vi "TIFF Read RGBA Image Oriented.vi"(0 "para0":cluster{}, 1 "para4":cluster{}, 5 "para1":cluster{}, 7 "para2":cluster{}, 9 "para3":cluster{}, 11 "error in (no error)":errorcluster, 12 "para5":cluster{}) -> (4 "para0 out":cluster{}, 6 "function return":i32, 10 "para3 out":cluster{}, 15 "error out":errorcluster)   [LabVIEW 2018]
doc: "LIBTIFF_DLL_IMPEXP int TIFFReadRGBAImageOriented(TIFF*, uint32, uint32, uint32*,\n int = ORIENTATION_BOTLEFT, int = 0);"
uses:
  libtiff3.dll
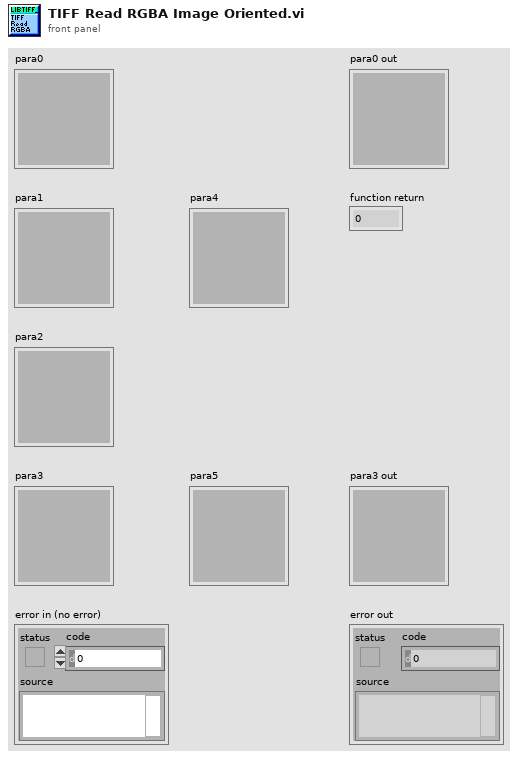
[diagram p1: front panel]
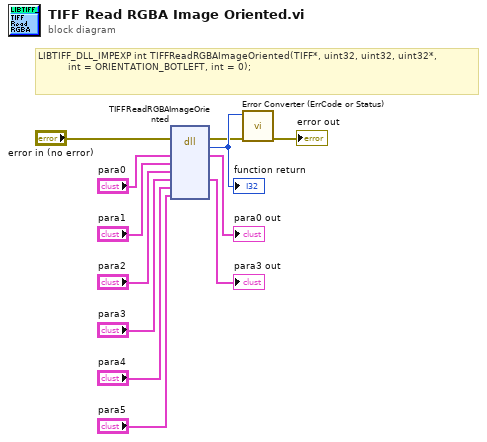
[diagram p0: block diagram]
diagram:
  # "LIBTIFF_DLL_IMPEXP\tint TIFFReadRGBAImageOriented(TIFF*, uint32, uint32, uint32*,\n\t\t\t\t      int = ORIENTATION_BOTLEFT, int = 0);"
  n1 = dll-call lib="C:/Users/johan/Downloads/LabVIEW software/LabVIEW software/IX-81 Software/lib/tiff/LibTiffLabview/libtiff3.*" fn="TIFFReadRGBAImageOriented"(error in="error in (no error)", "para0"="para0", "para1"="para1", "para2"="para2", "para3"="para3", "para4"="para4", "para5"="para5") -> (error out=w2:errorcluster, w12:i32, "para0"=→"para0 out":cluster{}, "para3"=→"para3 out":cluster{})  [unwired: 6 in, 1 out]
  "function return" <- w12
  n2 = call "Error Converter (ErrCode or Status).vi"("error in (no error)"=w2, "error code"=w12) -> ("error out"=→"error out":errorcluster)  [unwired: 9 in]
